vi "PAQmem_GetTimeRange.vi"(8 "error in (no error)":errorcluster, 11 "PAQ-memory in":refnum<class "PAQ-memory.lvclass">) -> (0 "error out":errorcluster, 1 "T_range":T1, 3 "PAQ-memory out":refnum<class "PAQ-memory.lvclass">)   [LabVIEW 2020, in "PAQ-memory.lvclass"]
doc: "Get the min and max time of the content of one memory layer"
uses:
  PAQ-memory.lvclass
  PAQ-memory.lvclass/PAQ-memory.ctl
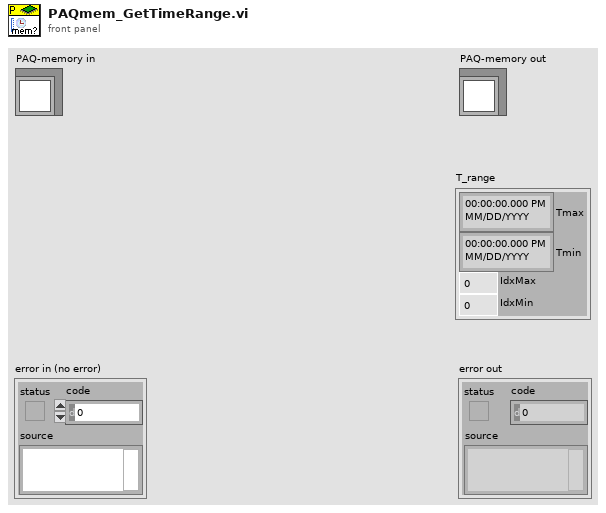
[diagram p1: front panel]
types:
  T1 = cluster{"Tmax":timestamp, "Tmin":timestamp, "IdxMax":i32, "IdxMin":i32}
  T2 = typedef "FAMM.lvclass/typedef_PAQdata.ctl" = cluster{"TAGs":string[], "Time":refnum<data-value>, "TAGdata":cluster{"source":refnum<data-value>, "status":refnum<data-value>, "data":refnum<data-value>, "max":refnum<data-value>, "min":refnum<data-value>}[]}
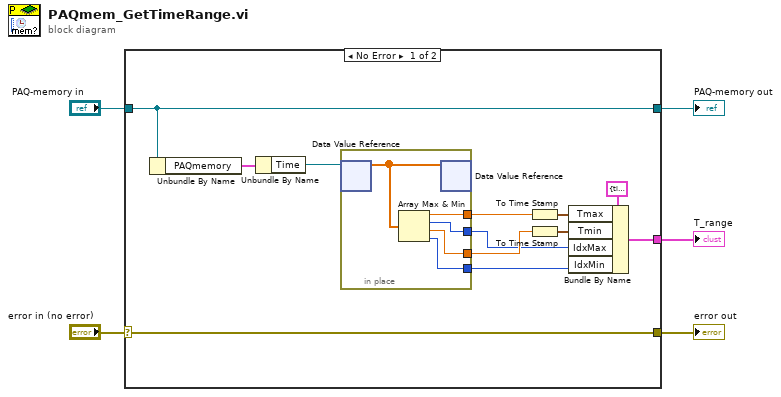
[diagram p0: block diagram]
diagram:
  n1 = case shown="No Error" "error in (no error)" {
    selector: "error in (no error)" -> [w17 w24]
    tunnel: [w17 w24] -> w4
    tunnel: [w16 w23] -> w2
    tunnel: "PAQ-memory in" -> [w16 w23]
    tunnel: [w12 _] -> w1
    frame No Error {
      n2 = Unbundle By Name(w16) -> ("PAQmemory"=w15:T2)
      n3 = Unbundle By Name(w15) -> ("Time"=w14:refnum<data-value>)
      n4 = in-place {
        in-place-border: [w21] -> w11
        in-place-border: [w20] -> w7
        in-place-border: [w19] -> w10
        in-place-border: [w18] -> w6
        n5 = in-place-dvr #1(w14) -> (w22:dbl[])  [unwired: 1 out]
        n6 = Array Max & Min(array=w22) -> (max value=w21:dbl, max index (indices)=w20:i32, min value=w19:dbl, min index (indices)=w18:i32)
        n7 = in-place-dvr #1(w22) -> ()  [unwired: 2 out]
      }
      n8 = To Time Stamp(1:w11) -> (0:w9:timestamp)
      n9 = To Time Stamp(1:w10) -> (0:w8:timestamp)
      n10 = Bundle By Name(cluster=T1 {"Tmax"=timestamp(0 s since 1904-01-01), "Tmin"=timestamp(0 s since 1904-01-01), "IdxMax"=0, "IdxMin"=0} ("T_range"), "Tmax"=w9, "Tmin"=w8, "IdxMax"=w7, "IdxMin"=w6) -> (w12:T1)
    }
    frame Error {
    }
  }
  "error out" <- w4
  "PAQ-memory out" <- w2
  "T_range" <- w1
